vi "Read Return FIFO.vi"(8 "error in (no error)":errorcluster, 9 "timeout in ms (0)":i32 format="%d ms", 11 "Transfer Group in":refnum<class "Transfer Group.lvclass">) -> (0 "error out":errorcluster, 1 "timed out?":bool, 2 "Transfer Group iteration":u64, 3 "Transfer Group out":refnum<class "Transfer Group.lvclass">)   [LabVIEW 2017, in "DSF Core.lvlib" / "Transfer Group.lvclass"]
uses:
  Transfer Group.lvclass
  Transfer Group.lvclass/Transfer Group.ctl
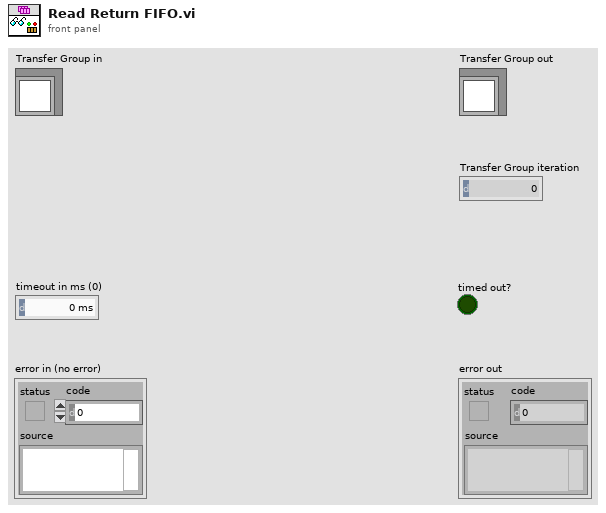
[diagram p1: front panel]
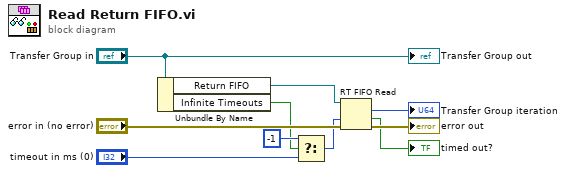
[diagram p0: block diagram]
diagram:
  n1 = Unbundle By Name("Transfer Group in") -> ("Return FIFO"=w1:refnum<k33>, "Infinite Timeouts"=w2:bool)
  n2 = Select(t=-1, s=w2, f="timeout in ms (0)") -> (s? t:f=w4:i32)
  n3 = RT FIFO Read(0:w1, 2:w4, 3:"error in (no error)") -> (9:→"Transfer Group iteration":u64, 10:→"timed out?":bool, 11:→"error out":errorcluster)  [unwired: 1 in, 2 out]
  "Transfer Group out" <- "Transfer Group in"
